vi "piezoDoubleWriteDynRegOpen.vi"   [LabVIEW 2017]
uses:
  globalDevices.vi
  <vilib>/DAQmx/create/channels.llb/DAQmx Create Channel (AO-Voltage-Basic).vi
  <vilib>/DAQmx/configure/timing.llb/DAQmx Timing (Sample Clock).vi
  <resource>/objmgr/daqmx.rc
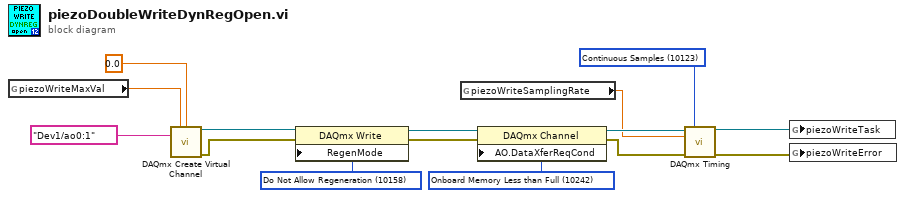
[diagram p0: block diagram]
diagram:
  w3 = 10123 items=["Finite Samples"=10178, "Continuous Samples"=10123, "Hardware Timed Single Point"=12522] ("sample mode")
  w7 = 10242 items=["Onboard Memory Empty"=10235, "Onboard Memory Half Full or Less"=10239, "Onboard Memory Less than Full"=10242] ("AO.DataXferReqCond")
  w10 = 10158 items=["Allow Regeneration"=10097, "Do Not Allow Regeneration"=10158] ("RegenMode")
  n1 = global read "globalDevices.vi" "piezoWriteMaxVal"() -> (w14:dbl)
  n2 = call-poly <vilib>:"DAQmx Create Virtual Channel.vi"("maximum value"=w14, "minimum value"=0.0, "physical channels"=tag "Dev1/ao0:1") -> ("task out"=w12:refnum<k21>, "error out"=w11:errorcluster)  [unwired: 11 in]
  n3 = property class="DAQmx Write"(reference=w12, error in=w11, "RegenMode"=w10) -> (reference out=w9:refnum<k21>, error out=w8:errorcluster)
  n4 = global read "globalDevices.vi" "piezoWriteSamplingRate"() -> (w4:dbl)
  n5 = property class="DAQmx Channel"(reference=w9, error in=w8, "AO.DataXferReqCond"=w7) -> (reference out=w6:refnum<k21>, error out=w5:errorcluster)
  n6 = call-poly <vilib>:"DAQmx Timing.vi"("task/channels in"=w6, "sample mode"=w3, "rate"=w4, "error in"=w5) -> ("task out"=w2:refnum<k21>, "error out"=w1:errorcluster)  [unwired: 10 in]
  n7 = global write "globalDevices.vi" "piezoWriteTask"(w2) -> ()
  n8 = global write "globalDevices.vi" "piezoWriteError"(w1) -> ()
